vi "ZLIB Store Stream__ogtk.vi"(4 "password (none)":string, 5 "local extra data":string, 6 "comment":string, 7 "global extra data":string, 8 "error in (no error)":errorcluster, 9 "internal name":string, 10 "source stream":string, 11 "zip Refnum":T2) -> (0 "error out":errorcluster, 3 "zip Refnum out":T2)   [LabVIEW 2011]
doc: "Adds a file to an archive in a zip session."
uses:
  <userlib>/_OpenG.lib/lvzip/lvzip.llb/ZLIB Zip Handle__ogtk.ctl
  <userlib>/_OpenG.lib/lvzip/lvzip.llb/ZLIB File Info__ogtk.ctl
panel:
  in  "file info":T1={"version"=0, "version needed"=0, "encrypted"=FALSE, "flag"=4294967295, "compression"=0, "dos date"=0, "crc"=0, "compressed size"=0, "uncompressed size"=0, "extra info"="", "file comment"="", "disk num start"=0, "internal fa"=0, "external fa"=0, "file timestamp"=0} {"file timestamp" format="%<%H:%M:%S\n%d/%m/%Y>T"; "external fa" format="%.0x"; "internal fa" format="%.0x"; "crc" format="%.0x"}
  # "Please visit http://www.OpenG.org to learn about the\nOpen Source LabVIEW software movement.\n\nNOTICE -- YOU MUST LEAVE THIS NOTICE IN PLACE.  PER THE TERMS OF THE LICENSE BELOW, YOU MAY SUBLICENSE THIS SOFTWARE \nIN ANY WAY THAT DOES NOT CONFLICT WITH THIS LICENSE.\n\n### BSD License (http://www.opensource.org/licenses/bsd-license.php) Begin ###\n \nCopyright (C) 2002-2004 Rolf Kalbermatter rolf.kalbermatter@citeng.com\nCopyright (C) 2002 Jim Kring jim@jimkring.com\n\nAll rights reserved.\n\nRedistribution and use in source and binary forms, with or without modification, are permitted provided that the following conditions are met:\n\n    * Redistributions of source code must retain the above copyright notice, this list of conditions and the following disclaimer.\n    * Redistributions in binary form must reproduce the above copyright notice, this list of conditions and the following disclaimer in the \n       documentation and/or other materials provided with the distribution.\n    * Neither the name of SciWare, James Kring, Inc., nor the names of its contributors may be used to endorse or promote products derived \n       from this software without specific prior written permission.\n\nTHIS SOFTWARE IS PROVIDED BY THE COPYRIGHT HOLDERS AND CONTRIBUTORS \"AS IS\" AND ANY EXPRESS OR IMPLIED WARRANTIES, \nINCLUDING, BUT NOT LIMITED TO, THE IMPLIED WARRANTIES OF MERCHANTABILITY AND FITNESS FOR A PARTICULAR PURPOSE ARE \nDISCLAIMED. IN NO EVENT SHALL THE COPYRIGHT OWNER OR CONTRIBUTORS BE LIABLE FOR ANY DIRECT, INDIRECT, INCIDENTAL,\n SPECIAL, EXEMPLARY, OR CONSEQUENTIAL DAMAGES (INCLUDING, BUT NOT LIMITED TO, PROCUREMENT OF SUBSTITUTE GOODS OR \nSERVICES; LOSS OF USE, DATA, OR PROFITS; OR BUSINESS INTERRUPTION) HOWEVER CAUSED AND ON ANY THEORY OF LIABILITY, \nWHETHER IN CONTRACT, STRICT LIABILITY, OR TORT (INCLUDING NEGLIGENCE OR OTHERWISE) ARISING IN ANY WAY OUT OF THE USE \nOF THIS SOFTWARE, EVEN IF ADVISED OF THE POSSIBILITY OF SUCH DAMAGE.\n\n### BSD License End ###"
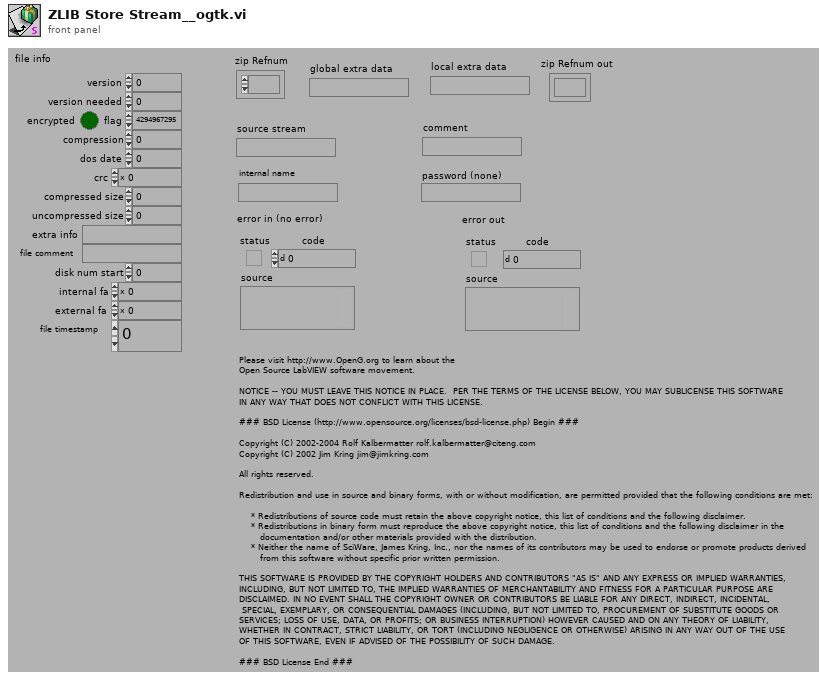
[diagram p1: front panel]
types:
  T1 = typedef "ZLIB File Info__ogtk.ctl" = cluster{"version":u32, "version needed":u32, "encrypted":bool, "flag":u32, "compression":i32, "dos date":u32, "crc":u32, "compressed size":u32, "uncompressed size":u32, "extra info":string, "file comment":string, "disk num start":u32, "internal fa":u32, "external fa":u32, "file timestamp":u32}
  T2 = typedef "ZLIB Zip Handle__ogtk.ctl" = refnum<k1>
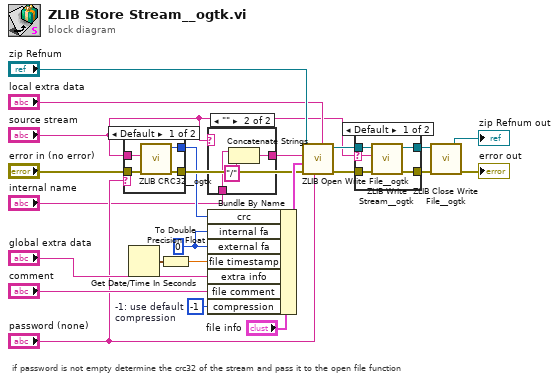
[diagram p0: block diagram]
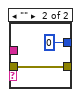
[diagram p2: hidden frame]
diagram:
  w5 = u32 0 ("internal fa")
  w8 = -1  # -1: use default compression
  # "if password is not empty determine the crc32 of the stream and pass it to the open file function"
  n1 = case shown="Default" "password (none)" {
    tunnel: "error in (no error)" -> [w27 w29]
    tunnel: [w24 w29] -> w10
    tunnel: [w25 u32 0 ("crc")] -> w9
    tunnel: "source stream" -> [w26 _]
    frame Default {
      n2 = call <userlib>:"ZLIB CRC32__ogtk.vi"("error in (no error)"=w27, "buffer"=w26) -> ("error out"=w24:errorcluster, "new crc32"=w25:u32)  [unwired: 4 in]
    }
    frame "" {
    }
  }
  n3 = Get Date/Time In Seconds() -> (seconds since 1Jan1904=w1:timestamp)
  n4 = To Double Precision Float(number=w1) -> (double precision float=w4:dbl)
  n5 = case shown="\"\"" "source stream" {
    tunnel: "internal name" -> [w30 w32]
    tunnel: [w30 w33] -> w17
    frame Default {
    }
    frame "" {
      n6 = Concatenate Strings(w32, "/" ("Format String")) -> (w33:string)
    }
  }
  n7 = Bundle By Name(cluster="file info", "crc"=w9, "internal fa"=w5, "external fa"=w5, "file timestamp"=w4, "extra info"="global extra data", "file comment"="comment", "compression"=w8) -> (w14:T1)
  n8 = call <userlib>:"ZLIB Open Write File__ogtk.vi"("local extra data"="local extra data", "password (none)"="password (none)", "error in (no error)"=w10, "file info"=w14, "filename"=w17, "zip Refnum"="zip Refnum") -> ("error out"=w21:errorcluster, "zip Refnum out"=w19:T2)  [unwired: 4 in]
  n9 = case shown="Default" "source stream" {
    selector: "source stream" -> [w34 _]
    tunnel: [w38 w39] -> w22
    tunnel: w21 -> [w37 w39]
    tunnel: w19 -> [w36 w40]
    tunnel: [w35 w40] -> w18
    frame Default {
      n10 = call <userlib>:"ZLIB Write Stream__ogtk.vi"("error in (no error)"=w37, "byte stream"=w34, "zip Refnum"=w36) -> ("error out"=w38:errorcluster, "zip Refnum out"=w35:T2)  [unwired: 4 in]
    }
    frame "" {
    }
  }
  n11 = call <userlib>:"ZLIB Close Write File__ogtk.vi"("error in (no error)"=w22, "zip Refnum"=w18) -> ("error out"=→"error out":errorcluster, "zip Refnum out"=→"zip Refnum out":T2)  [unwired: 4 in]
